vi "vipPublish.vi"() -> (0 "error out":errorcluster)   [LabVIEW 2014, in "lv-cli-steps.lvlib"]
uses:
  lv-cli-steps.lvlib
  <vilib>/Utility/error.llb/DialogType.ctl
  <vilib>/Wiresmith Technology/LabVIEW CLI/CLI Class/CLI.lvclass
  <vilib>/JKI/VIPM API/VIPM API_vipm_api.lvlib
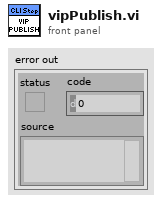
[diagram p1: front panel]
types:
  T1 = typedef "DialogType.ctl" = u16
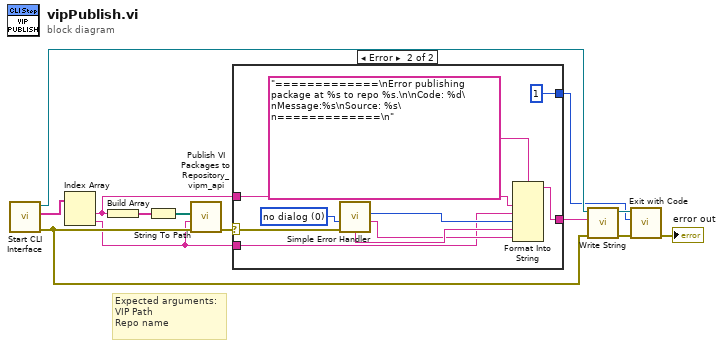
[diagram p0: block diagram]
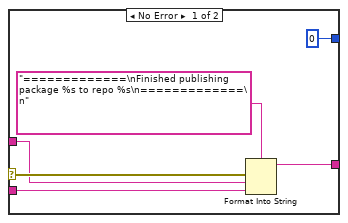
[diagram p2: hidden frame]
diagram:
  # "Expected arguments:\nVIP Path\nRepo name"
  n1 = call <vilib>:"Start CLI Interface.vi"() -> ("error out"=w4:errorcluster, "Custom Parameters"=w13:string[], "CLI out"=w11:refnum<class "CLI.lvclass">)  [unwired: 9 in]
  n2 = Index Array(array=w13) -> (element #1=w6:string, element #2=w1:string)  [unwired: 2 in]
  n3 = Build Array(w6) -> (w3:string[])
  n4 = String To Path(string=w3) -> (path=w2:path[])
  n5 = call <vilib>:"Publish VI Packages to Repository_vipm_api.vi"("error in (no error)"=w4, "Repository Name"=w1, "Packages to publish to Repository Library (vip,ogp)"=w2) -> ("error out"=w5:errorcluster)  [unwired: 7 in, 1 out]
  n6 = case shown="Error" w5 {
    selector: w5 -> [w18 w28]
    tunnel: w6 -> [w17 w24]
    tunnel: [w16 w29] -> w12
    tunnel: [0 ("Exit Code (0)") 1 ("Exit Code (0)")] -> w8
    tunnel: w1 -> [w14 w20]
    frame No Error {
      n7 = Format Into String(format string="=============\nFinished publishing package %s to repo %s\n=============\n", error in=w18, w17, w14) -> (resulting string=w16:string)  [unwired: 1 in, 1 out]
    }
    frame Error {
      w27 = T1 0 items=["no dialog", "OK message", "continue or stop message", "OK message + warnings", "continue/stop + warnings"] ("type of dialog (OK msg:1)")
      n8 = call <vilib>:"Simple Error Handler.vi"("type of dialog (OK msg:1)"=w27, "error in (no error)"=w28) -> ("code out"=w21:i32, "source out"=w22:string, "message"=w23:string)  [unwired: 3 in, 2 out]
      n9 = Format Into String(format string="=============\nError publishing package at %s to repo %s.\n\nCode: %d\nMessage:%s\nSource: %s\n=============\n", w24, w20, w21, w23, w22) -> (resulting string=w29:string)  [unwired: 2 in, 1 out]
    }
  }
  n10 = call <vilib>:"Write String.vi"("error in (no error)"=w4, "Text to Write"=w12, "CLI in"=w11) -> ("error out"=w10:errorcluster, "CLI out"=w9:refnum<class "CLI.lvclass">)  [unwired: 7 in]
  n11 = call <vilib>:"Exit with Code.vi"("error in (no error)"=w10, "Exit Code (0)"=w8, "CLI in"=w9) -> ("error out"=→"error out":errorcluster)  [unwired: 8 in]
